vi "Clean_rawdata.vi"(8 "error in (no error)":errorcluster caption="entrée d'erreur (pas d'erreur)", 9 "N of scans":i32, 10 "Data RAW in":u32[][](array[numeric]), 11 "VIS-NIR en entrée":refnum<class "VIS-NIR.lvclass">) -> (0 "error out":errorcluster caption="sortie d'erreur", 1 "I 2":i32[][](array[numeric]), 2 "I":i32[][](array[numeric]), 3 "VIS-NIR en sortie":refnum<class "VIS-NIR.lvclass">, 4 "II RAW":i32[](array[numeric]))   [LabVIEW 2015, in "VIS-NIR.lvclass"]
uses:
  VIS-NIR.lvclass
panel:
  in  "Zeros/Up_down":bool=TRUE
  in  "exchange I and II":bool
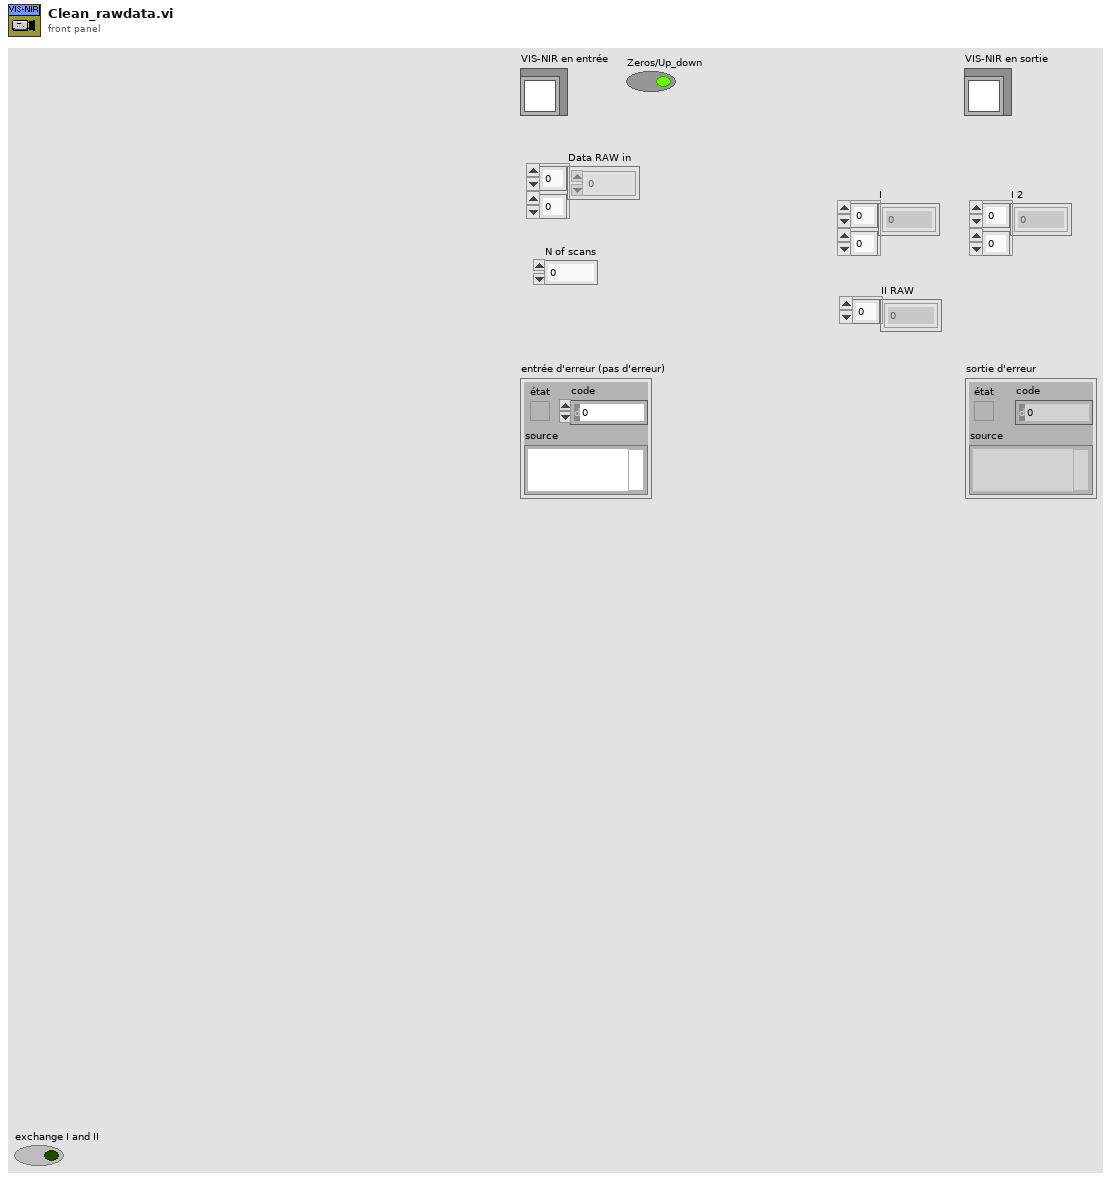
[diagram p1: front panel]
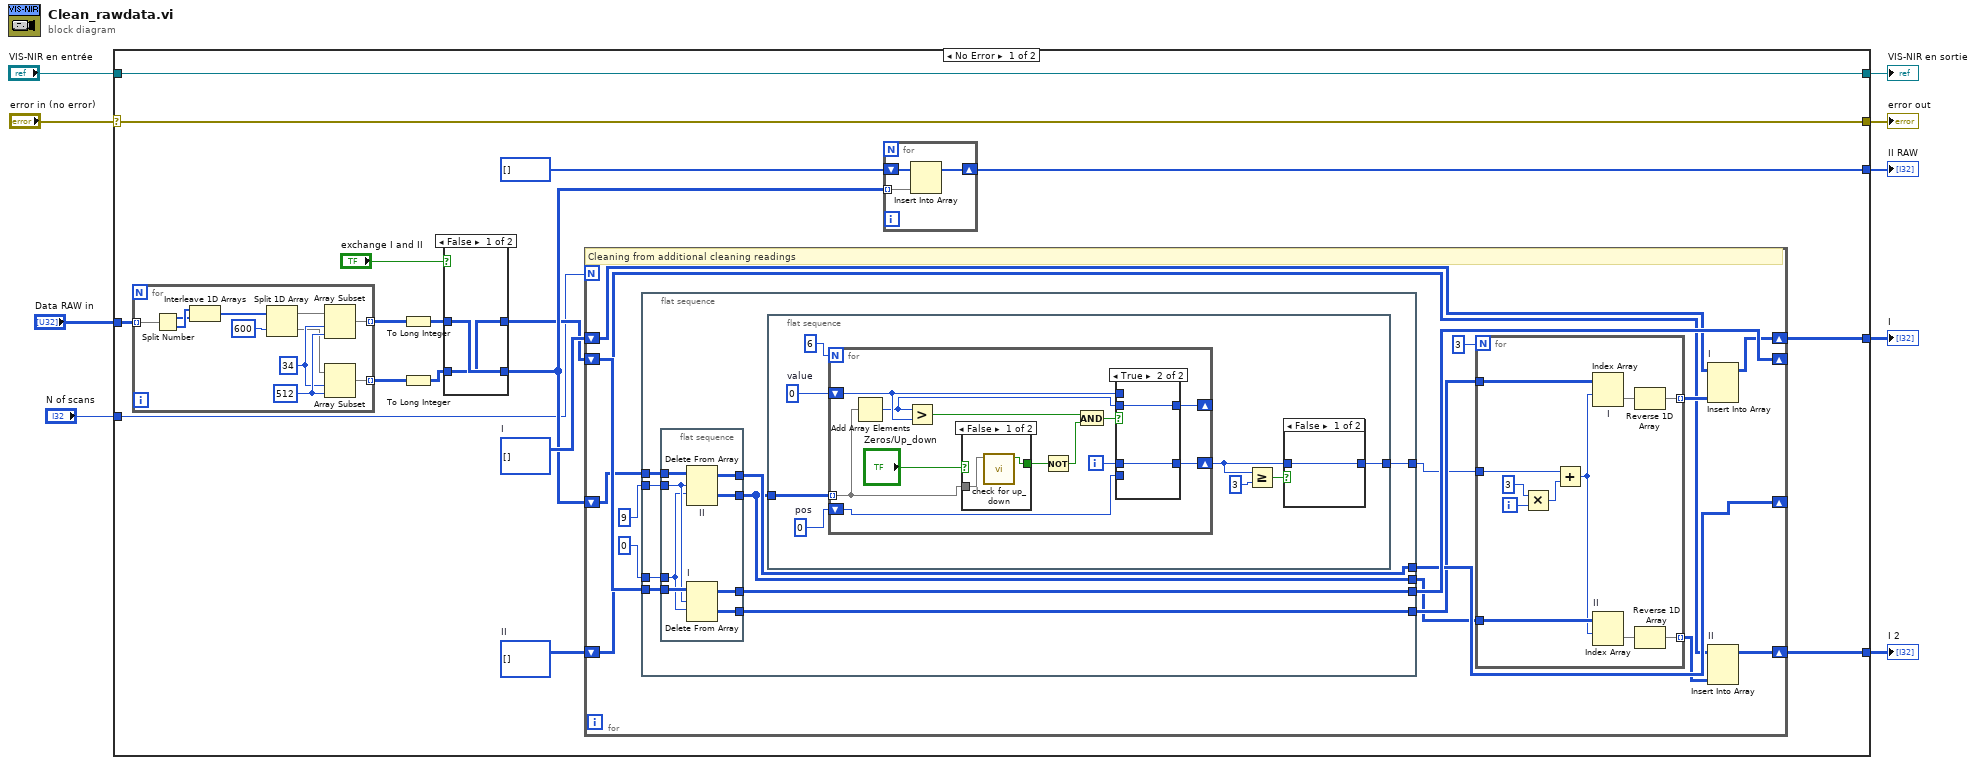
[diagram p0: block diagram]
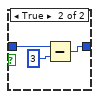
[diagram p2: hidden frame]
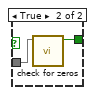
[diagram p3: hidden frame]
diagram:
  n1 = case shown="No Error" "error in (no error)" {
    selector: "error in (no error)" -> [w15 w122]
    tunnel: [w15 w122] -> w8
    tunnel: [w26 w121] -> w6
    tunnel: "VIS-NIR en entrée" -> [w26 w121]
    tunnel: [w14 _] -> w5
    tunnel: [w13 _] -> w4
    tunnel: [w12 _] -> w3
    tunnel: "Data RAW in" -> [w11 _]
    tunnel: "N of scans" -> [w10 _]
    frame No Error {
      w25 = i32[][] []  # II
      w24 = i32[][] []  # I
      n2 = for {
        tunnel: [w106] -> w20 mode=indexing
        tunnel: [w107] -> w22 mode=indexing
        tunnel: w11 -> [w105] mode=indexing
        w110 = 34 ("indice")
        w111 = 512 ("longueur")
        n3 = Split Number(x=w105) -> (hi(x)=w103:u16[], lo(x)=w104:u16[])
        n4 = Interleave 1D Arrays(w104, w103) -> (w113:u16[])
        n5 = Split 1D Array(array=w113, index=600 ("indice")) -> (first subarray=w109:u16[], second subarray=w108:u16[])
        n6 = Array Subset(array=w109, index=w110, length=w111) -> (w106:u16[])
        n7 = Array Subset(array=w108, index=w110, length=w111) -> (w107:u16[])
      }
      n8 = To Long Integer(number=w20) -> (32bit integer=w21:i32[][])
      n9 = To Long Integer(number=w22) -> (32bit integer=w23:i32[][])
      n10 = case shown="False" "exchange I and II" {
        tunnel: [w114 w117] -> w17
        tunnel: w21 -> [w115 w117]
        tunnel: w23 -> [w114 w116]
        tunnel: [w115 w116] -> w18
        frame False {
        }
        frame True {
        }
      }
      n11 = for {
        N: w10 -> [_]
        shift-right: [w41] -> _
        shift-left: w17 -> [w42]
        shift-right: [w39] -> _
        shift-left: w18 -> [w40]
        shift-right: [w30] -> w14
        shift-left: w24 -> [w31]
        shift-right: [w27] -> w13
        shift-left: w25 -> [w28]
        # "Cleaning from additional cleaning readings"
        n12 = flat-sequence {
          tunnel: w42 -> [w51]
          tunnel: [w50] -> w41
          tunnel: w40 -> [w49]
          tunnel: [w48] -> w39
          tunnel: 9 ("length") -> [w47]
          tunnel: 0 ("index (row)") -> [w46]
          tunnel: [w45] -> w36
          tunnel: [w44] -> w35
          tunnel: [w43] -> w34
          frame #0 {
            n13 = flat-sequence {
              tunnel: w51 -> [w91]
              tunnel: [w90] -> w50
              tunnel: w49 -> [w89]
              tunnel: [w88] -> w48
              tunnel: w47 -> [w87]
              tunnel: w46 -> [w86]
              tunnel: [w85] -> w45
              tunnel: [w84] -> w44
              frame #0 {
                n14 = Delete From Array "II"(array=w89, length=w87, index (row)=w86) -> (deleted portion=w84:i32[][], array with subset deleted=w88:i32[][])  [unwired: 1 in]
                n15 = Delete From Array "I"(array=w91, length=w87, index (row)=w86) -> (deleted portion=w85:i32[][], array with subset deleted=w90:i32[][])  [unwired: 1 in]
              }
            }
            n16 = flat-sequence {
              tunnel: w44 -> [w53]
              tunnel: [w52] -> w43
              frame #0 {
                w57 = 0  # pos
                w58 = 0  # value
                n17 = for {
                  N: 6 -> [_]
                  tunnel: w53 -> [w65] mode=indexing
                  shift-right: [w75] -> _
                  shift-left: w58 -> [w74]
                  shift-right: [w70] -> w55
                  shift-left: w57 -> [w72]
                  i -> [w71]
                  n18 = Add Array Elements(numeric array=w65) -> (sum=w73:i32)
                  n19 = Greater?(x=w73, y=w74) -> (0:w69:bool)
                  n20 = case shown="False" "Zeros/Up_down" {
                    tunnel: [w76 w79] -> w68
                    tunnel: w65 -> [w77 w78]
                    frame False {
                      n21 = call "check for up_down.vi"("Array"=w77) -> ("Yes/No"=w76:bool)  [unwired: 10 in]
                    }
                    frame True {
                      n22 = call "check for zeros.vi"("Array"=w78) -> ("Yes/No"=w79:bool)  [unwired: 10 in]
                    }
                  }
                  n23 = Not(x=w68) -> (.not. x?=w66:bool)
                  n24 = And(x=w69, y=w66) -> (x .and. y?=w67:bool)
                  n25 = case shown="True" w67 {
                    tunnel: [w81 w83] -> w75
                    tunnel: w74 -> [w81 _]
                    tunnel: w73 -> [_ w83]
                    tunnel: [w80 w82] -> w70
                    tunnel: w72 -> [w80 _]
                    tunnel: w71 -> [_ w82]
                    frame False {
                    }
                    frame True {
                    }
                  }
                }
                n26 = Greater Or Equal?(x=w55, y=3) -> (x >= y?=w54:bool)
                n27 = case shown="False" w54 {
                  tunnel: [w60 w61] -> w52
                  tunnel: w55 -> [w60 w63]
                  frame False {
                  }
                  frame True {
                    n28 = Subtract(x=w63, y=3) -> (x-y=w61:i32)
                  }
                }
              }
            }
          }
        }
        n29 = for {
          N: 3 -> [_]
          tunnel: w36 -> [w102]
          tunnel: w35 -> [w101]
          tunnel: w34 -> [w97]
          tunnel: [w92] -> w32 mode=indexing
          tunnel: [w94] -> w29 mode=indexing
          i -> [w100]
          n30 = Multiply(x=3, y=w100) -> (x*y=w98:i32)
          n31 = Add(x=w97, y=w98) -> (x+y=w96:i32)
          n32 = Index Array "I"(array=w102, index (row)=w96) -> (element=w93:i32[])  [unwired: 1 in]
          n33 = Index Array "II"(array=w101, index (row)=w96) -> (element=w95:i32[])  [unwired: 1 in]
          n34 = Reverse 1D Array(array=w93) -> (reversed array=w92:i32[])
          n35 = Reverse 1D Array(array=w95) -> (reversed array=w94:i32[])
        }
        n36 = Insert Into Array "I"(array=w31, new element=w32) -> (w30:i32[][])  [unwired: 2 in]
        n37 = Insert Into Array "II"(array=w28, new element=w29) -> (w27:i32[][])  [unwired: 2 in]
      }
      n38 = for {
        tunnel: w18 -> [w119] mode=indexing
        shift-right: [w118] -> w12
        shift-left: i32[] [] ("II RAW") -> [w120]
        n39 = Insert Into Array(array=w120, new element=w119) -> (w118:i32[])  [unwired: 1 in]
      }
    }
    frame Error {
    }
  }
  "error out" <- w8
  "VIS-NIR en sortie" <- w6
  "I" <- w5
  "I 2" <- w4
  "II RAW" <- w3
